vi "Main.vi"(8 "error in (no error)":errorcluster, 11 "Thread in":refnum<class "Thread.lvclass">) -> (0 "error out":errorcluster, 3 "Thread out":refnum<class "Thread.lvclass">)   [LabVIEW 2019, in "DSF Core.lvlib" / "Thread.lvclass"]
uses:
  Thread.lvclass
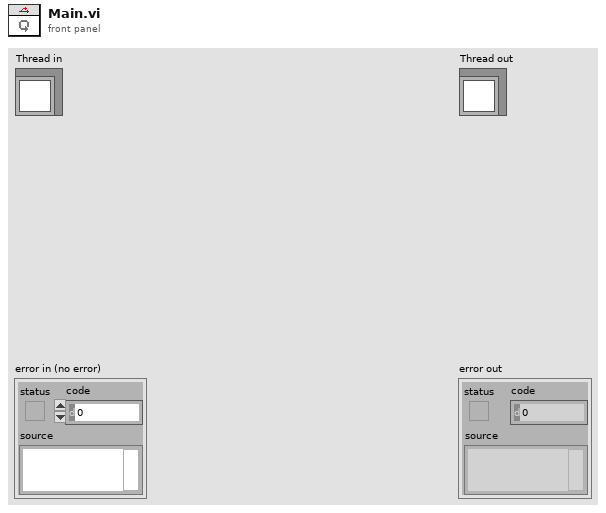
[diagram p1: front panel]
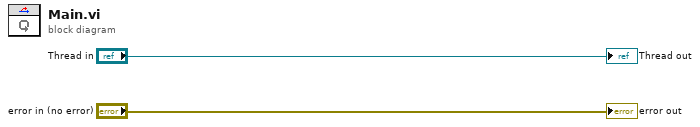
[diagram p0: block diagram]
diagram:
  "error out" <- "error in (no error)"
  "Thread out" <- "Thread in"
